vi "Run Test.vi"(8 "error in (no error)":errorcluster, 11 "Test Template in":refnum<class "Instrument Close.lvclass">) -> (0 "error out":errorcluster, 1 "Positions":i32[](array[numeric]), 2 "Tests Passed":bool[](array[boolean]), 3 "Test Template out":refnum<class "Instrument Close.lvclass">, 5 "Fail Codes":string[](array[string]))   [LabVIEW 2015, in "Instrument Close.lvclass"]
uses:
  Instrument Close.lvclass
  CBTF Applications/Driver Board Testing/Main/Application/Application/Class/typedefs/Instrument Selector -- Enum.ctl
  Test Class/Test Class.lvclass/Test Class.ctl
  Classes/Application/Class/Application.lvclass
  Test Class/Test Class.lvclass
  CBTF Applications/Driver Board Testing/Main/Application/Application/Class/Driver Board Test.lvclass
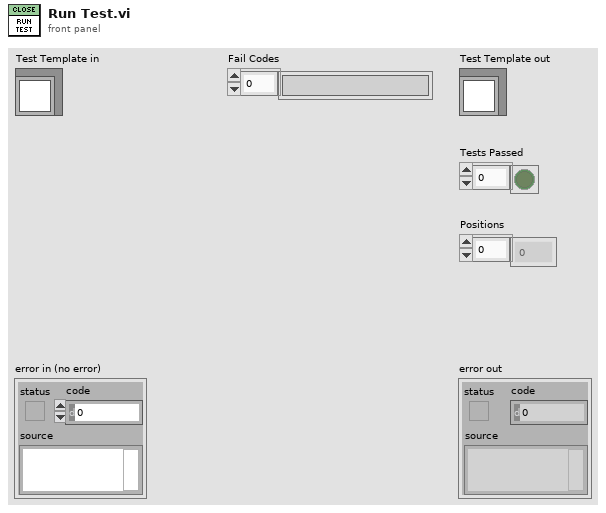
[diagram p1: front panel]
types:
  T1 = typedef "Driver Board Test.lvlib/Driver Board Test.lvclass/Instrument Selector -- Enum.ctl" = enum16{"ACPS1", "ACPS2", "DCPS1", "DCPS2", "DCPS3", "DCLoad1", "DCLoad2", "DPM1", "DPM2", "Switch1", "PXI1Slot2", "PXI1Slot3", "cDAQ1Mod5", "cDAQ1Mod6", "cDAQ1Mod7", "cDAQ1Mod8", "cDAQ1Mod1", "cDAQ1Mod2", "cDAQ1Mod3", "cDAQ1Mod4", "cDAQ2Mod1", "cDAQ2Mod2", "cDAQ2Mod3", "cDAQ2Mod4"}
  T2 = typedef "Application.lvlib/App Properties.lvclass/Class Properties -- Cluster.ctl" = cluster{"UUT Info":T3[], "Test Information":refnum<vi>, "Test Complete Event":refnum<user-event>, "Shop Floor System":refnum<class "Shop Floor System.lvclass">, "Gold Board":refnum<class "Golden Board.lvclass">, "Test Recipe":refnum<class "Test Recipe.lvclass">, "Instruments":refnum<class "Instrument.lvclass">[], "Mode":T4, "Test Results":T5[], "Station Config":refnum<class "Station Config.lvclass">}
  T3 = typedef "Application.lvlib/App Properties.lvclass/UUT Reference -- Cluster.ctl" = cluster{"Serial Number Reference":refnum<vi>, "Status Message Reference":refnum<vi>}
  T4 = typedef "Application.lvlib/Application.lvclass/Op Mode -- Enum.ctl" = u16
  T5 = typedef "Application.lvlib/App Properties.lvclass/Test Result -- Cluster.ctl" = cluster{"Position":i32, "Pass":bool, "Fail Codes":string}
  T6 = cluster{"Serial Number Reference":refnum<vi>, "Status Message Reference":refnum<vi>, "Position":u32}[]
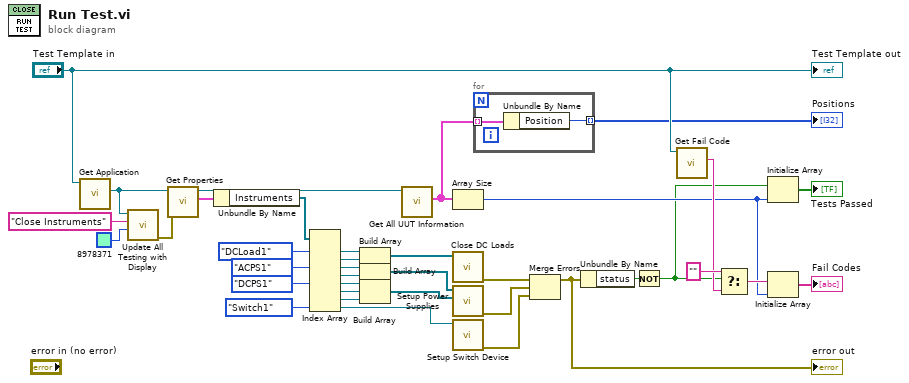
[diagram p0: block diagram]
diagram:
  n1 = call "Get Application.vi"("Test Class in"="Test Template in") -> ("Application.lvlib:Application.lvclass"=w10:refnum<class "Application.lvclass">)  [unwired: 9 in, 1 out]
  n2 = call "Update All Testing with Display.vi"("BG Color"=u32 8978371, "Message ('')"="Close Instruments", "Application in"=w10) -> ("error out"=w8:errorcluster)  [unwired: 7 in, 1 out]
  n3 = call "Get Properties.vi"("error in (no error)"=w8, "Acrobat Template in"=w10) -> ("Class Properties"=w37:T2, "Acrobat Template out"=w5:refnum<class "Application.lvclass">)  [unwired: 7 in, 1 out]
  n4 = Unbundle By Name(w37) -> ("Instruments"=w36:refnum<class "Instrument.lvclass">[])
  n5 = Index Array(array=w36, index #1=Instrument_Selector_--_Enum."DCLoad1" ("Instrument"), index #3=Instrument_Selector_--_Enum."ACPS1" ("Instrument"), index #5=Instrument_Selector_--_Enum."DCPS1" ("Instrument"), index #8=Instrument_Selector_--_Enum."Switch1" ("Instrument")) -> (element #1=w26:refnum<class "Instrument.lvclass">, element #2=w25:refnum<class "Instrument.lvclass">, element #3=w28:refnum<class "Instrument.lvclass">, element #4=w27:refnum<class "Instrument.lvclass">, element #5=w17:refnum<class "Instrument.lvclass">, element #6=w16:refnum<class "Instrument.lvclass">, element #7=w15:refnum<class "Instrument.lvclass">, element #8=w12:refnum<class "Instrument.lvclass">)  [unwired: 4 in]
  n6 = Build Array(w26, w25) -> (w21:refnum<class "Instrument.lvclass">[])
  n7 = Build Array(w28, w27) -> (w14:refnum<class "Instrument.lvclass">[])
  n8 = Build Array(w17, w16, w15) -> (w13:refnum<class "Instrument.lvclass">[])
  n9 = call-dynamic "Get All UUT Information.vi"("Application in"=w5) -> ("Active UUTs"=w2:T6)  [unwired: 8 in, 2 out]
  n10 = Array Size(array=w2) -> (size(s)=w4:i32)
  n11 = call "Close DC Loads.vi"("DC Loads"=w21) -> ("Error out"=w34:errorcluster)  [unwired: 10 in]
  n12 = call "Setup Power Supplies.vi"("DC Supplies"=w13, "AC Supplies"=w14) -> ("error out"=w24:errorcluster)  [unwired: 9 in]
  n13 = call "Setup Switch Device.vi"("Instrument in"=w12) -> ("error out"=w23:errorcluster)  [unwired: 10 in]
  n14 = for {
    tunnel: w2 -> [w39] mode=indexing
    tunnel: [w38] -> w1 mode=indexing
    n15 = Unbundle By Name(w39) -> ("Position"=w38:u32)
  }
  "Positions" <- w1
  n16 = Merge Errors(w34, w24, w23) -> (w22:errorcluster)
  "error out" <- w22
  n17 = Unbundle By Name(w22) -> ("status"=w33:bool)
  n18 = Not(x=w33) -> (.not. x?=w3:bool)
  n19 = call "Get Fail Code.vi"("Test Class in"="Test Template in") -> ("Fail Code"=w30:string)  [unwired: 9 in, 1 out]
  n20 = Select(t="", s=w3, f=w30) -> (s? t:f=w31:string)
  n21 = Initialize Array(w3, w4) -> (→"Tests Passed":bool[])
  n22 = Initialize Array(w31, w4) -> (→"Fail Codes":string[])
  "Test Template out" <- "Test Template in"
